vi "testSDOBatch.vi"() -> ()   [LabVIEW 2013]
uses:
  <vilib>/CANopenLib/CANOPEN.llb/CANopen BaudRate.ctl
  <vilib>/CANopenLib/CANOPEN.llb/CANopen Interface Create.vi
  <vilib>/CANopenLib/CANOPEN.llb/CANopen SDO Create.vi
  <vilib>/CANopenLib/CANOPEN.llb/CANopen SDO Close.vi
  <vilib>/CANopenLib/CANOPEN.llb/CANopen Interface Close.vi
panel:
  out "completion code":u32
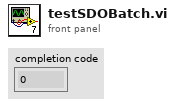
[diagram p1: front panel]
types:
  T1 = typedef "CANopen BaudRate.ctl" = u32
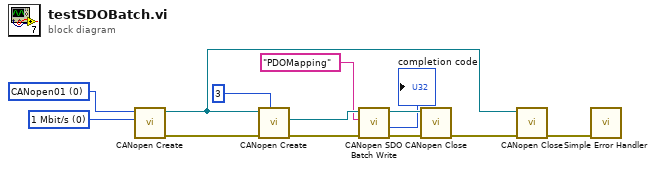
[diagram p0: block diagram]
diagram:
  w12 = T1 0 items=["1 Mbit/s"=0, "800 kbit/s"=1, "500 kbit/s"=2, "250 kbit/s"=3, "125 kbit/s"=4, "50 kbit/s"=6, "20 kbit/s"=7, "10 kbit/s"=8] ("baud rate")
  w13 = u32 0 items=["CANopen01", "CANopen02", "CANopen03", "CANopen04", "CANopen05", "CANopen06", "CANopen07", "CANopen08", "CANopen09", "CANopen10", "CANopen11", "CANopen12", "CANopen13", "CANopen14", "CANopen15", "CANopen16", "CANopen17", "CANopen18", "CANopen19", "CANopen20", "CANopen21", "CANopen22", "CANopen23", "CANopen24", "CANopen25", "CANopen26", "CANopen27", "CANopen28", "CANopen29", "CANopen30", "CANopen31", "CANopen32"] ("interface name")
  n1 = call-poly <vilib>:"CANopen Create.vi"("baud rate"=w12, "interface name"=w13) -> ("error out"=w3:errorcluster, "interface object out"=w8:refnum<k20>)  [unwired: 8 in]
  n2 = call-poly <vilib>:"CANopen Create.vi"("node-ID"=u8 3, "error in (no error)"=w3, "interface object in"=w8) -> ("error out"=w4:errorcluster, "SDO object out"=w10:refnum<k20>)  [unwired: 6 in, 1 out]
  n3 = call <vilib>:"CANopen SDO Batch Write.vi"("error in (no error)"=w4, "batch SDO name"="PDOMapping", "SDO object in"=w10) -> ("error out"=w6:errorcluster, "completion code"=→"completion code":u32, "SDO object out"=w9:refnum<k20>)  [unwired: 6 in]
  n4 = call-poly <vilib>:"CANopen Close.vi"("error in (no error)"=w6, "SDO object in"=w9) -> ("error out"=w7:errorcluster)  [unwired: 9 in]
  n5 = call-poly <vilib>:"CANopen Close.vi"("error in (no error)"=w7, "interface object in"=w8) -> ("error out"=w2:errorcluster)  [unwired: 9 in]
  n6 = call <vilib>:"Simple Error Handler.vi"("error in (no error)"=w2) -> ()  [unwired: 4 in, 5 out]
